vi "Scale RGB Channels Demo.vi"() -> ()   [LabVIEW 2012, in "Picture Box Tools.lvlib"]
uses:
  Picture Box Tools.lvlib
panel:
  out "Scale Picture":picture caption="已修改图片"
  out "Origin Picture":picture caption="源图片"
  in  "Scale":cluster{"Red":dbl, "Green":dbl, "Blue":dbl} {"Blue" scale=0.0..100.0; "Green" scale=0.0..100.0; "Red" scale=0.0..100.0}
  in  "停止按钮":bool
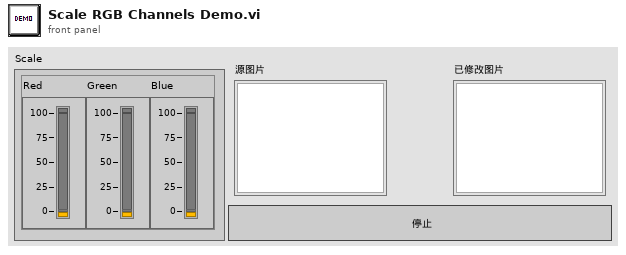
[diagram p1: front panel]
types:
  T1 = typedef "imagedata.ctl" = cluster{"image type":i32, "image depth":i32, "image":u8[], "mask":u8[], "colors":u32[], "Rectangle":cluster{"left":i16, "top":i16, "right":i16, "bottom":i16}}
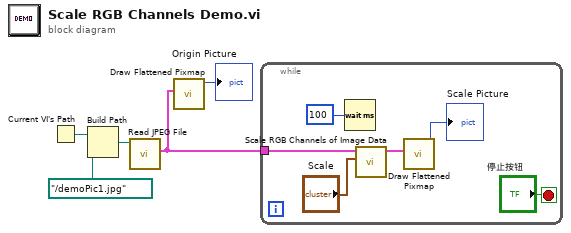
[diagram p0: block diagram]
diagram:
  n1 = Current VI's Path() -> (path=w3:path)
  n2 = Build Path(base path=w3, name or relative path=path "../demoPic1.jpg") -> (appended path=w5:path)
  n3 = call <vilib>:"Read JPEG File.vi"("path to JPEG file"=w5) -> ("image data"=w1:T1)  [unwired: 8 in, 2 out]
  n4 = call <vilib>:"Draw Flattened Pixmap.vi"("image data"=w1) -> ("new picture"=→"Origin Picture":picture)  [unwired: 8 in]
  n5 = while {
    tunnel: w1 -> [w9]
    stop <- "停止按钮" stop-if-true
    n6 = Wait (ms)(milliseconds to wait=u32 100 ("等待时间（毫秒）")) -> ()  [unwired: 1 out]
    n7 = call "Scale RGB Channels of Image Data.vi"("Scale"="Scale", "image data In"=w9) -> ("image data Out"=w6:T1)  [unwired: 8 in, 1 out]
    n8 = call <vilib>:"Draw Flattened Pixmap.vi"("image data"=w6) -> ("new picture"=→"Scale Picture":picture)  [unwired: 8 in]
  }
